vi "Write_Trace_Database.vi"   [LabVIEW 2013]
uses:
  <vilib>/lvdsc/historical/Open Trace (Numeric).vi
  <vilib>/lvdsc/historical/Write Trace (Numeric).vi
  <vilib>/lvdsc/historical/Read Trace (Numeric).vi
  <vilib>/lvdsc/NI_DSC.lvlib
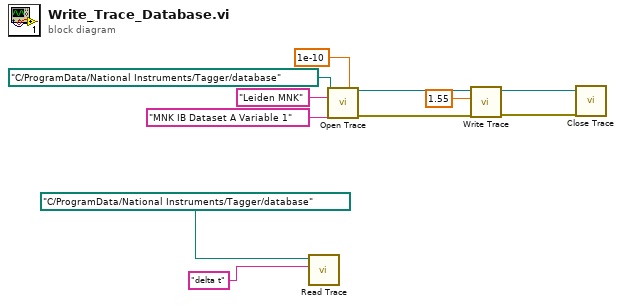
[diagram p0: block diagram]
diagram:
  n1 = call-poly <vilib>:"Read Trace.vi"("trace name"="delta t" ("regular expression"), "database URL"=path "C:/ProgramData/National Instruments/Tagger/database") -> ()  [unwired: 6 in, 4 out]
  n2 = call-poly <vilib>:"Open Trace.vi"("database URL"=path "C:/ProgramData/National Instruments/Tagger/database", "value precision (0.01)"=1e-10, "process name"="Leiden MNK", "trace name"="MNK IB Dataset A Variable 1") -> ("trace reference"=w10:refnum<k1>, "error out"=w4:errorcluster)  [unwired: 9 in, 1 out]
  n3 = call-poly <vilib>:"Write Trace.vi"("error in (no error)"=w4, "value"=1.55, "trace ref"=w10) -> ("error out"=w3:errorcluster, "trace ref out"=w11:refnum<k1>)  [unwired: 7 in]
  n4 = call <vilib>:"Close Trace.vi"("error in (no error)"=w3, "trace reference"=w11) -> ()  [unwired: 9 in, 1 out]
